vi "drawobj.vi"(10 "new picture in":picture, 11 "Digital in":refnum<vi>) -> (3 "new picture out":picture)   [LabVIEW 2016]
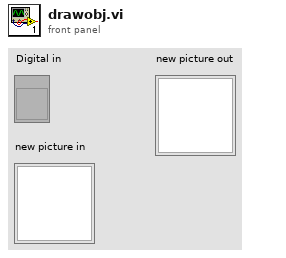
[diagram p1: front panel]
types:
  T1 = cluster{"Width":u16, "Style":enum32{"Solid", "Dash", "Dot", "DashDot", "DashDotDot"}}
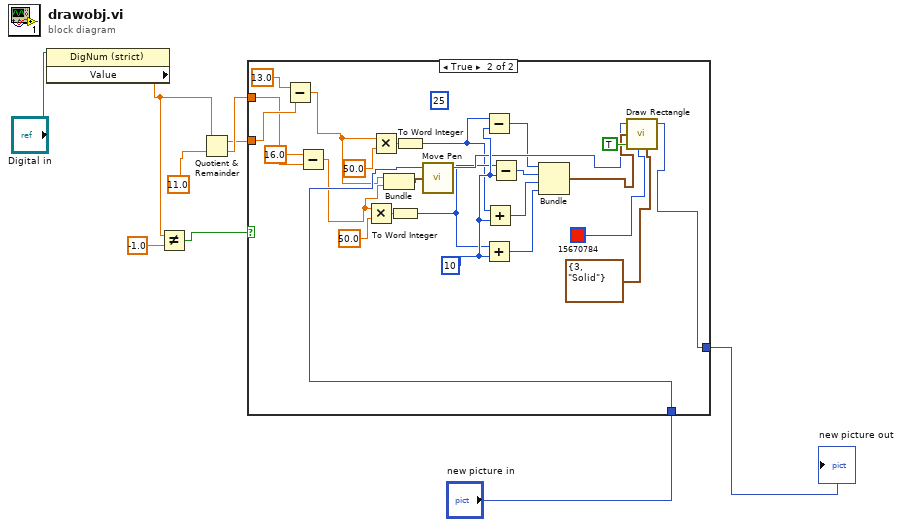
[diagram p0: block diagram]
diagram:
  n1 = property class="DigNum (strict)"(reference="Digital in") -> ("Value"=w2:dbl)  [unwired: 1 in, 2 out]
  n2 = Not Equal?(x=w2, y=-1.0) -> (x != y?=w3:bool)
  n3 = Quotient & Remainder(x=w2, y=11.0) -> (x-y*floor(x/y)=w4:dbl, floor(x/y)=w5:dbl)
  n4 = case shown="True" w3 {
    tunnel: [w10 w30] -> w9
    tunnel: "new picture in" -> [w10 w28]
    tunnel: w5 -> [_ w11]
    tunnel: w4 -> [_ w12]
    frame False {
    }
    frame True {
      w35 = 10
      (unwired) i16 25 ("Waypoint \nSize")
      n5 = Subtract(x=13.0, y=w12) -> (x-y=w15:dbl)
      n6 = Subtract(x=16.0, y=w11) -> (x-y=w13:dbl)
      n7 = Multiply(x=w13, y=50.0) -> (x*y=w24:dbl)
      n8 = Multiply(x=w15, y=50.0) -> (x*y=w22:dbl)
      n9 = Bundle(w15, w13) -> (w27:cluster{dbl, dbl})  [unwired: 1 in]
      n10 = To Word Integer(number=w24) -> (16bit integer=w26:i16)
      n11 = To Word Integer(number=w22) -> (16bit integer=w23:i16)
      n12 = call <vilib>:"Move Pen.vi"("new position"=w27, "picture"=w28) -> ("new picture"=w29:picture)  [unwired: 3 in]
      n13 = Subtract(x=w23, y=w35) -> (x-y=w17:i32)
      n14 = Add(x=w26, y=w35) -> (x+y=w20:i32)
      n15 = Add(x=w23, y=w35) -> (x+y=w19:i32)
      n16 = Subtract(x=w26, y=w35) -> (x-y=w18:i32)
      n17 = Bundle(w17, w18, w19, w20) -> (w31:cluster{i32, i32, i32, i32})  [unwired: 1 in]
      n18 = call <vilib>:"Draw Rectangle.vi"("picture"=w29, "rect"=w31, "fill?(F)"=TRUE, "color(black)"=u32 15670784, "pen"=T1 {"Width"=3, "Style"=enum."Solid"}) -> ("new picture"=w30:picture)  [unwired: 4 in]
    }
  }
  "new picture out" <- w9
